vi "get_vector.vi"() -> ()   [LabVIEW 2015]
panel:
  out "Sigma":dbl
  out "Average":dbl
  out "Array":dbl[](array[numeric])
  in  "File Path Control":path
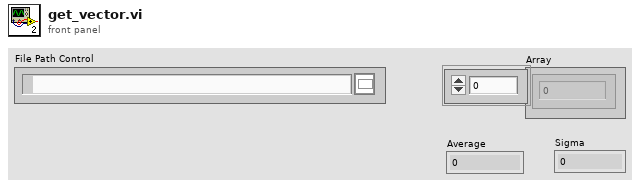
[diagram p1: front panel]
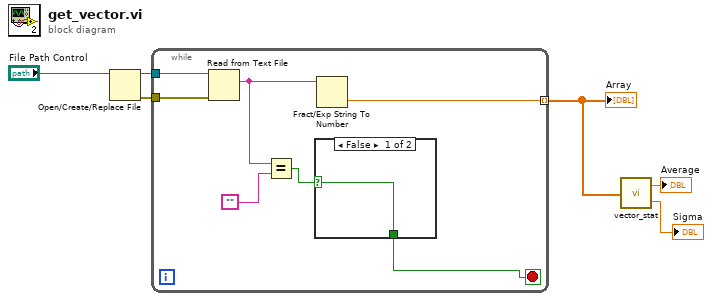
[diagram p0: block diagram]
diagram:
  n1 = Open/Create/Replace File(file path (use dialog)="File Path Control") -> (refnum out=w5:refnum<file>, error out=w4:errorcluster)  [unwired: 5 in, 1 out]
  n2 = while {
    tunnel: w5 -> [w13]
    tunnel: w4 -> [w12]
    tunnel: [w11] -> w3 mode=indexing
    stop <- w7 stop-if-true
    n3 = Read from Text File(file (use dialog)=w13, error in=w12) -> (text=w9:string)  [unwired: 2 in, 3 out]
    n4 = Equal?(x=w9, y="") -> (x = y?=w10:bool)
    n5 = case shown="False" w10 {
      selector: w10 -> [w14 w15]
      tunnel: [w14 w15] -> w7
      frame False {
      }
      frame True {
      }
    }
    n6 = Fract/Exp String To Number(string=w9) -> (number=w11:dbl)  [unwired: 3 in, 1 out]
  }
  "Array" <- w3
  n7 = call "vector_stat.vi"("Array"=w3) -> ("Average"=→"Average":dbl, "Sigma"=→"Sigma":dbl)
